vi "Accelerometer.vi"(8 "Error In":errorcluster, 11 "Serial Port":refnum<visa-resource-name>="COM4") -> (0 "Error Out":errorcluster)   [LabVIEW 2015]
uses:
  <vilib>/MakerHub/LINX/Private/Type Defs/User Platform.ctl
  <vilib>/MakerHub/LINX/Private/Type Defs/Interface.ctl
  <vilib>/MakerHub/LINX/Public/Peripherals/Analog/Analog Read 1 Chan.vi
  <vilib>/MakerHub/LINX/LMH-LINX.lvlib
panel:
  in  "stop":bool
  out "Waveform Chart":i16(graph)
  out "Numeric":i32
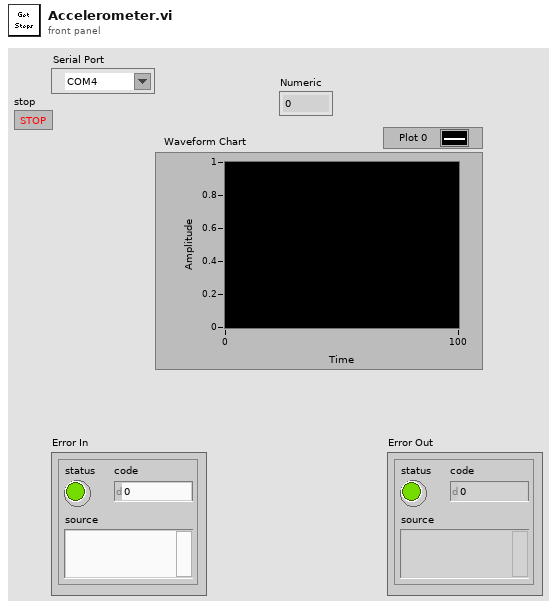
[diagram p1: front panel]
types:
  T1 = typedef "LMH-LINX.lvlib/Interface.ctl" = enum16{"Serial", "TCP"}
  T2 = typedef "LMH-LINX.lvlib/User Platform.ctl" = enum16{"Default", "LINX", "myRIO"}
  T3 = typedef "LMH-LINX.lvlib/LINX Ref.ctl" = cluster{"Platform":T4, "Interface":T1, "LINX Device Config":T5}
  T4 = typedef "LMH-LINX.lvlib/Platform.ctl" = enum16{"LINX", "myRIO"}
  T5 = typedef "LMH-LINX.lvlib/Device.lvlib/LINX Device Config.ctl" = cluster{"Interface":T1, "COM Port":refnum<visa-resource-name>, "TCP Configuration":T6, "Device Family":u8, "Device ID":u8, "Device Name":string, "TCP Ref":refnum<k5>, "Channels":T7}
  T6 = typedef "LMH-LINX.lvlib/Device.lvlib/TCP Config.ctl" = cluster{"IP Address":string, "Port":u16}
  T7 = typedef "LMH-LINX.lvlib/Channels.ctl" = cluster{"DI":u8[], "DO":u8[], "AI":u8[], "AO":u8[], "PWM":u8[], "QE":u8[], "UART":u8[], "I2C 2":u8[], "SPI":u8[], "CAN":u8[], "Servo":u8[], "AI Ref (V)":dbl, "AO Ref (V)":dbl, "AO Resolution (Bits)":u8}
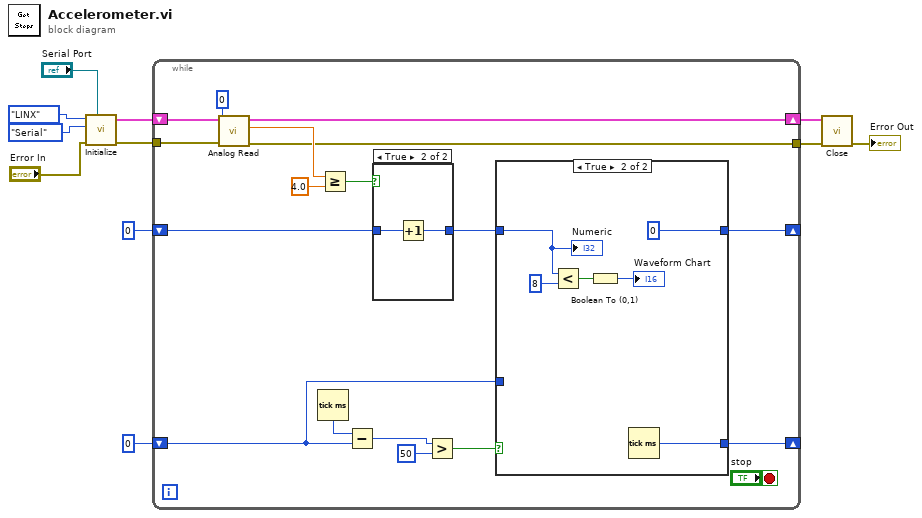
[diagram p0: block diagram]
diagram:
  n1 = call <vilib>:"Initialize.vi"("Serial Port"="Serial Port", "Error In"="Error In", "Interface"=Interface."Serial", "Platform"=User_Platform."LINX") -> ("Error Out"=w4:errorcluster, "LINX Ref"=w8:T3)  [unwired: 5 in, 1 out]
  n2 = while {
    shift-right: [w28] -> w7
    shift-left: w8 -> [w29]
    shift-right: [w17] -> _
    shift-left: 0 -> [w23]
    shift-right: [w15] -> _
    shift-left: 0 -> [w16]
    tunnel: w4 -> [w14]
    tunnel: [w13] -> w3
    stop <- "stop" stop-if-true
    n3 = call-poly <vilib>:"Analog Read.vi"("Error In"=w14, "Analog Channel"=u8 0, "LINX Resource"=w29) -> ("Error Out"=w13:errorcluster, "AI Value"=w26:dbl, "LINX Resource"=w28:T3)  [unwired: 5 in, 1 out]
    n4 = Tick Count (ms)() -> (millisecond timer value=w22:u32)
    n5 = Greater Or Equal?(x=w26, y=4.0) -> (x >= y?=w24:bool)
    n6 = Subtract(x=w22, y=w16) -> (x-y=w21:u32)
    n7 = case shown="True" w24 {
      tunnel: w23 -> [w38 w40]
      tunnel: [w38 w39] -> w18
      frame False {
      }
      frame True {
        n8 = Increment(x=w40) -> (x+1=w39:i32)
      }
    }
    n9 = Greater?(x=w21, y=u32 50) -> (0:w19:bool)
    n10 = case shown="True" w19 {
      tunnel: w18 -> [w31 w35]
      tunnel: [w31 0] -> w17
      tunnel: w16 -> [w30 _]
      tunnel: [w30 w36] -> w15
      frame False {
      }
      frame True {
        n11 = Less?(x=w35, y=8) -> (x < y?=w33:bool)
        n12 = Boolean To (0,1)(Boolean=w33) -> (0, 1=→"Waveform Chart":i16)
        n13 = Tick Count (ms)() -> (millisecond timer value=w36:u32)
        "Numeric" <- w35
      }
    }
  }
  n14 = call <vilib>:"Close.vi"("Error In"=w3, "LINX Resource"=w7) -> ("Error Out"=→"Error Out":errorcluster)  [unwired: 8 in, 1 out]
